vi "PORT_DIR.vi"(2 "error in (no error)":errorcluster, 3 "PIOs directions":i8=1 min=0 max=63 step=1 format="%x", 4 "read/write":dbl=1.0 min=0.0 max=1.0, 5 "VISA resource Input":refnum<visa-resource-name>) -> (0 "error out":errorcluster, 1 "VISA resource name out":refnum<visa-resource-name>)   [LabVIEW 2011]
panel:
  out "unsigned byte array":u8[](array[numeric])
  out "x+y":dbl
  out "Read PORT command":u8[](array[numeric])
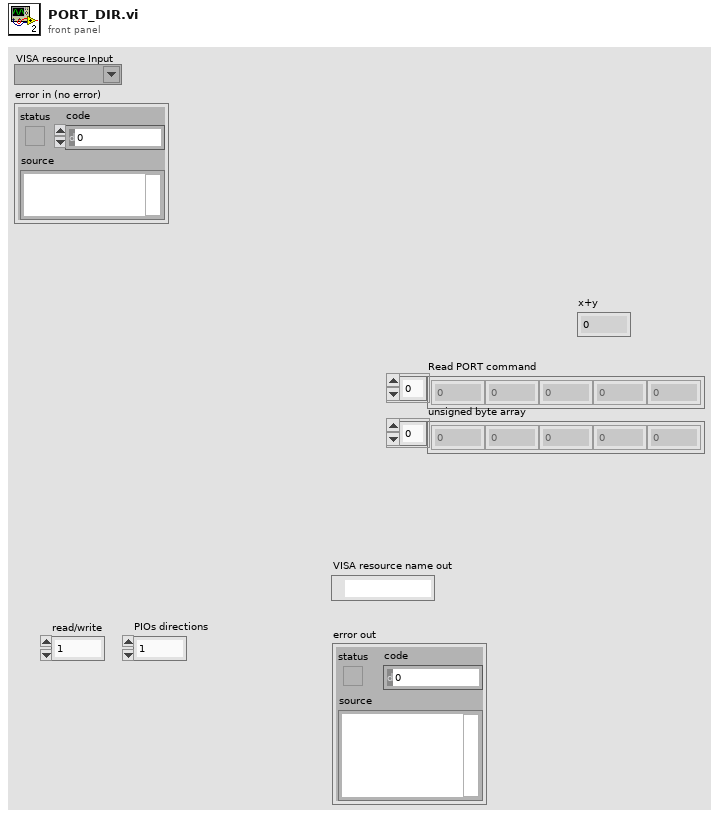
[diagram p1: front panel]
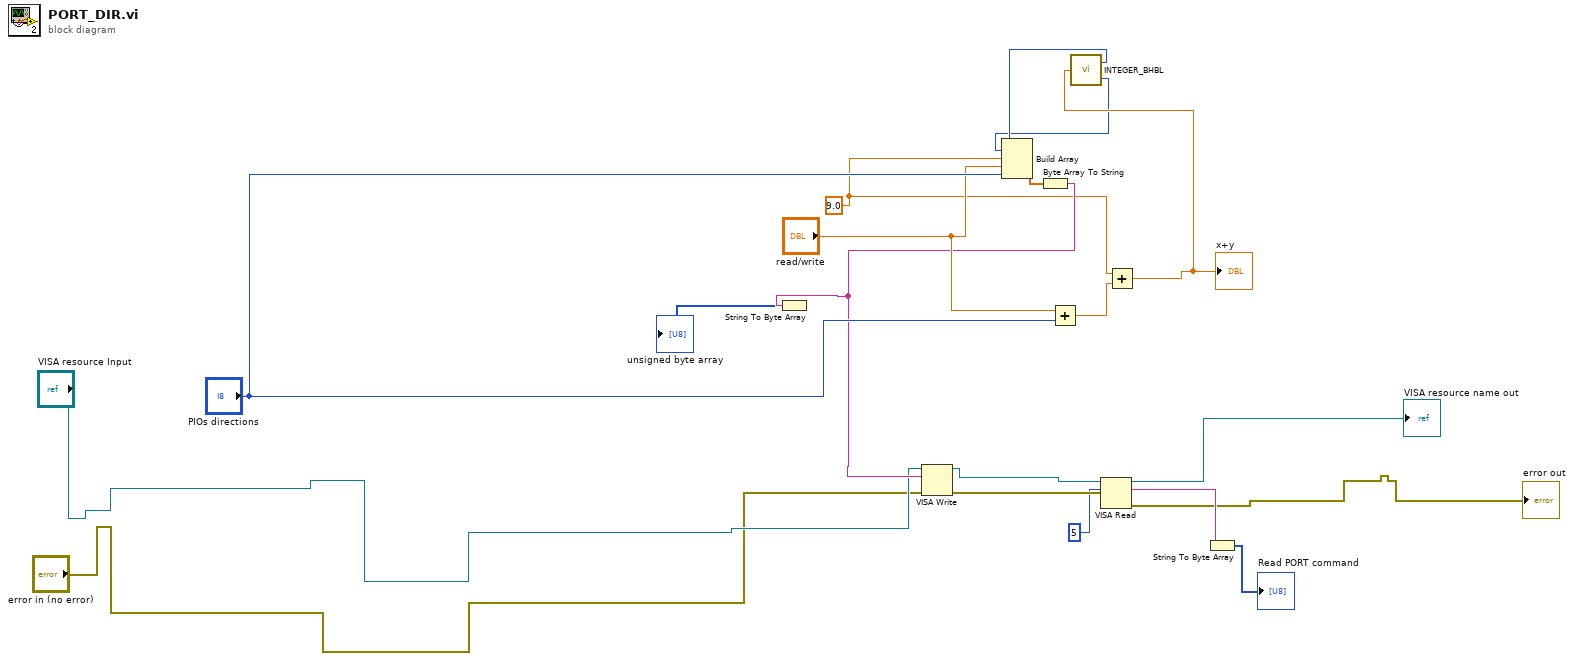
[diagram p0: block diagram]
diagram:
  w4 = 9.0 ("element")
  n1 = Add(x="read/write", y="PIOs directions") -> (x+y=w11:dbl)
  n2 = Add(x=w4, y=w11) -> (x+y=w10:dbl)
  "x+y" <- w10
  n3 = call "INTEGER_BHBL.vi"("int16"=w10) -> ("Lvalue"=w8:u8, "HValue"=w9:u8)
  n4 = Build Array(w9, w8, w4, "read/write", "PIOs directions") -> (w14:dbl[])
  n5 = Byte Array To String(unsigned byte array=w14) -> (string=w7:string)
  n6 = String To Byte Array(string=w7) -> (unsigned byte array=→"unsigned byte array":u8[])
  n7 = VISA Write(VISA resource name="VISA resource Input", write buffer=w7, error in (no error)="error in (no error)") -> (VISA resource name out=w15:refnum<visa-resource-name>, error out=w16:errorcluster)  [unwired: 1 out]
  n8 = VISA Read(VISA resource name=w15, byte count=u32 5, error in (no error)=w16) -> (VISA resource name out=→"VISA resource name out":refnum<visa-resource-name>, read buffer=w18:string, error out=→"error out":errorcluster)  [unwired: 1 out]
  n9 = String To Byte Array(string=w18) -> (unsigned byte array=→"Read PORT command":u8[])
